vi "Send Autosampler Prime Pump.vi"(5 "Cycles":u16=5, 6 "Correlation ID":u32, 7 "Message Priority (Normal)":T1=enum."Normal", 8 "error in (no error)":errorcluster, 9 "Waste Valve Pos.":u16=2, 10 "Buffer Val Pos.":u16=3, 11 "Message Enqueuer":refnum<class "Message Enqueuer.lvclass">) -> (0 "error out":errorcluster, 3 "Message Enqueuer out":refnum<class "Message Enqueuer.lvclass">)   [LabVIEW 2023, in "Application.lvlib" / "Autosampler Prime Pump Msg.lvclass"]
doc: "This VI sends the message to an actor."
uses:
  Autosampler Prime Pump Msg.lvclass
  <vilib>/ActorFramework/Message Enqueuer/Message Enqueuer.lvclass
  <vilib>/ActorFramework/Message Enqueuer/Message Priority.ctl
  C:/Program Files/National Instruments/LabVIEW 2023/vi.lib/ActorFramework/Message/Message.lvclass
  Autosampler Prime Pump Msg.lvclass/Autosampler Prime Pump Msg.ctl
  <vilib>/ActorFramework/Message Enqueuer/Message Enqueuer.lvclass/Message Enqueuer.ctl
  <vilib>/ActorFramework/Message Priority Queue/Priority Enqueue.vi
  C:/FLASH/Development/Application Messages/Autosampler Prime Pump Msg/Autosampler Prime Pump Msg.lvclass
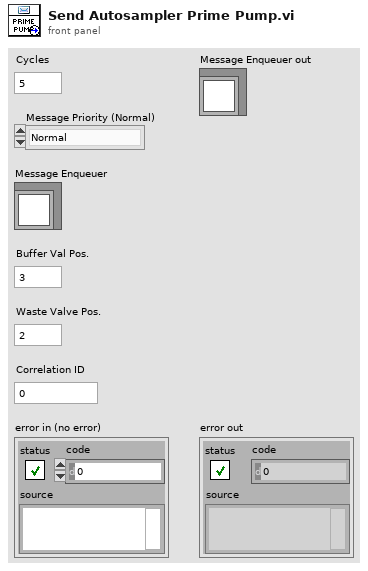
[diagram p1: front panel]
types:
  T1 = typedef "Actor Framework.lvlib/Message Enqueuer.lvclass/Message Priority.ctl" = enum16{"Low", "Normal", "High"}
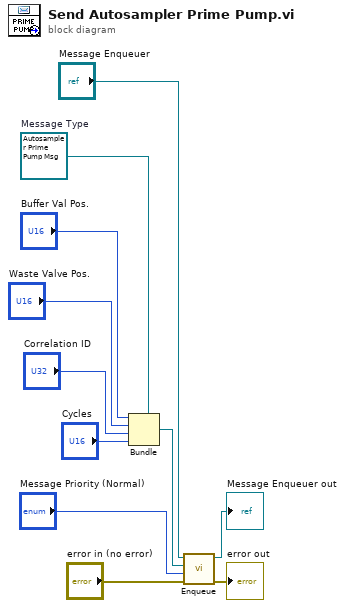
[diagram p0: block diagram]
diagram:
  w8 = refnum<class "Autosampler Prime Pump Msg.lvclass"> refnum  # Message Type
  n1 = Bundle(cluster=w8, "Buffer Val Pos.", "Waste Valve Pos.", "Correlation ID", "Cycles") -> (w7:refnum<class "Autosampler Prime Pump Msg.lvclass">)
  n2 = call <vilib>:"Enqueue.vi"("error in (no error)"="error in (no error)", "Message Priority (Normal)"="Message Priority (Normal)", "Message"=w7, "Message Enqueuer in"="Message Enqueuer") -> ("error out"=→"error out":errorcluster, "Message Enqueuer in"=→"Message Enqueuer out":refnum<class "Message Enqueuer.lvclass">)  [unwired: 6 in]
